vi "Run Tests (TestSuite Object Array).vi"(7 "TextTestRunner in":refnum<class "TextTestRunner.lvclass">, 8 "error in (no error)":errorcluster, 10 "TestCase Objects":refnum<class "TestSuite.lvclass">[](array[class])) -> (0 "error out":errorcluster, 1 "test details":string, 2 "successful?":bool)   [LabVIEW 2011, in "VI Tester API.lvlib"]
doc: "Run TestSuite objects."
uses:
  VI Tester API.lvlib
  Classes/TestSuite/TestSuite.lvclass
  Classes/TextTestRunner/TextTestRunner.lvclass
panel:
  # "JKI VI Tester for LabVIEW\nhttp://jkisoft.com/vi-tester\nCopyright (C) 2007-2009, JKI <info@jkisoft.com>\nALL RIGHTS RESERVED"
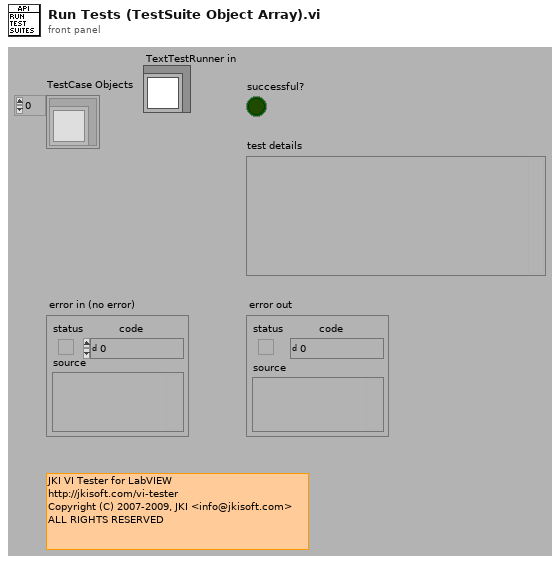
[diagram p1: front panel]
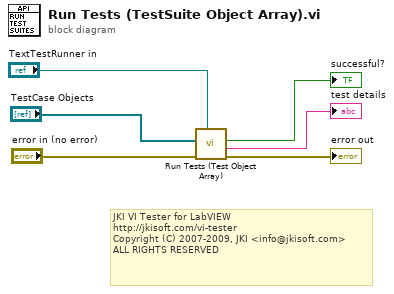
[diagram p0: block diagram]
diagram:
  # "JKI VI Tester for LabVIEW\nhttp://jkisoft.com/vi-tester\nCopyright (C) 2007-2009, JKI <info@jkisoft.com>\nALL RIGHTS RESERVED"
  n1 = call "Run Tests (Test Object Array).vi"("TextTestRunner in"="TextTestRunner in", "error in (no error)"="error in (no error)", "Tests"="TestCase Objects") -> ("error out"=→"error out":errorcluster, "test details"=→"test details":string, "successful?"=→"successful?":bool)  [unwired: 6 in]
